vi "0926New Project.vi"() -> ()   [LabVIEW 2011] (continued)
\n7783468750.000000#-39.000000#-4.400000#-18.000000#-10.000000#-3.000000#-30.000000#-30.000000\r\n7789712500.000000#-39.000000#-4.400000#-18.000000#-10.000000#-3.000000#-30.000000#-30.000000\r\n7795956250.000000#-39.000000#-4.400000#-18.000000#-10.000000#-3.000000#-30.000000#-30.000000\r\n7802200000.000000#-39.000000#-4.400000#-18.000000#-10.000000#-3.000000#-30.000000#-30.000000\r\n7808443750.000000#-39.000000#-4.400000#-18.000000#-10.000000#-3.000000#-30.000000#-30.000000\r\n7814687500.000000#-39.000000#-4.400000#-18.000000#-10.000000#-3.000000#-30.000000#-30.000000\r\n7820931250.000000#-39.000000#-4.400000#-18.000000#-10.000000#-3.000000#-30.000000#-30.000000\r\n7827175000.000000#-39.000000#-4.400000#-18.000000#-10.000000#-3.000000#-30.000000#-30.000000\r\n7833418750.000000#-39.000000#-4.400000#-18.000000#-10.000000#-3.000000#-30.000000#-30.000000\r\n7839662500.000000#-39.000000#-4.400000#-18.000000#-10.000000#-3.000000#-30.000000#-30.000000\r\n7845906250.000000#-39.000000#-4.400000#-18.000000#-10.000000#-3.000000#-30.000000#-30.000000\r\n7852150000.000000#-39.000000#-4.400000#-18.000000#-10.000000#-3.000000#-30.000000#-30.000000\r\n7858393750.000000#-39.000000#-4.400000#-18.000000#-10.000000#-3.000000#-30.000000#-30.000000\r\n7864637500.000000#-39.000000#-4.400000#-18.000000#-10.000000#-3.000000#-30.000000#-30.000000\r\n7870881250.000000#-39.000000#-4.400000#-18.000000#-10.000000#-3.000000#-30.000000#-30.000000\r\n7877125000.000000#-39.000000#-4.400000#-18.000000#-10.000000#-3.000000#-30.000000#-30.000000\r\n7883368750.000000#-39.000000#-4.400000#-18.000000#-10.000000#-3.000000#-30.000000#-30.000000\r\n7889612500.000000#-39.000000#-4.400000#-18.000000#-10.000000#-3.000000#-30.000000#-30.000000\r\n7895856250.000000#-39.000000#-4.400000#-18.000000#-10.000000#-3.000000#-30.000000#-30.000000\r\n7902100000.000000#-39.000000#-4.400000#-18.000000#-10.000000#-3.000000#-30.000000#-30.000000\r\n7908343750.000000#-39.000000#-4.400000#-18.000000#-10.000000#-3.000000#-30.000000#-30.000000\r\n7914587500.000000#-39.000000#-4.400000#-18.000000#-10.000000#-3.000000#-30.000000#-30.000000\r\n7920831250.000000#-39.000000#-4.400000#-18.000000#-10.000000#-3.000000#-30.000000#-30.000000\r\n7927075000.000000#-39.000000#-4.400000#-18.000000#-10.000000#-3.000000#-30.000000#-30.000000\r\n7933318750.000000#-39.000000#-4.400000#-18.000000#-10.000000#-3.000000#-30.000000#-30.000000\r\n7939562500.000000#-39.000000#-4.400000#-18.000000#-10.000000#-3.000000#-30.000000#-30.000000\r\n7945806250.000000#-39.000000#-4.400000#-18.000000#-10.000000#-3.000000#-30.000000#-30.000000\r\n7952050000.000000#-39.000000#-4.400000#-18.000000#-10.000000#-3.000000#-30.000000#-30.000000\r\n7958293750.000000#-39.000000#-4.400000#-18.000000#-10.000000#-3.000000#-30.000000#-30.000000\r\n7964537500.000000#-39.000000#-4.400000#-18.000000#-10.000000#-3.000000#-30.000000#-30.000000\r\n7970781250.000000#-39.000000#-4.400000#-18.000000#-10.000000#-3.000000#-30.000000#-30.000000\r\n7977025000.000000#-39.000000#-4.400000#-18.000000#-10.000000#-3.000000#-30.000000#-30.000000\r\n7983268750.000000#-39.000000#-4.400000#-18.000000#-10.000000#-3.000000#-30.000000#-30.000000\r\n7989512500.000000#-39.000000#-4.400000#-18.000000#-10.000000#-3.000000#-30.000000#-30.000000\r\n7995756250.000000#-39.000000#-4.400000#-18.000000#-10.000000#-3.000000#-30.000000#-30.000000\r\n8002000000.000000#-39.000000#-4.400000#-18.000000#-10.000000#-3.000000#-30.000000#-30.000000\r\n8008243750.000000#-39.000000#-4.400000#-18.000000#-10.000000#-3.000000#-30.000000#-30.000000\r\n8014487500.000000#-39.000000#-4.400000#-18.000000#-10.000000#-3.000000#-30.000000#-30.000000\r\n8020731250.000000#-39.000000#-4.400000#-18.000000#-10.000000#-3.000000#-30.000000#-30.000000\r\n8026975000.000000#-39.000000#-4.400000#-18.000000#-10.000000#-3.000000#-30.000000#-30.000000\r\n8033218750.000000#-39.000000#-4.400000#-18.000000#-10.000000#-3.000000#-30.000000#-30.000000\r\n8039462500.000000#-39.000000#-4.400000#-18.000000#-10.000000#-3.000000#-30.000000#-30.000000\r\n8045706250.000000#-39.000000#-4.400000#-18.000000#-10.000000#-3.000000#-30.000000#-30.000000\r\n8051950000.000000#-39.000000#-4.400000#-18.000000#-10.000000#-3.000000#-30.000000#-30.000000\r\n8058193750.000000#-39.000000#-4.400000#-18.000000#-10.000000#-3.000000#-30.000000#-30.000000\r\n8064437500.000000#-39.000000#-4.400000#-18.000000#-10.000000#-3.000000#-30.000000#-30.000000\r\n8070681250.000000#-39.000000#-4.400000#-18.000000#-10.000000#-3.000000#-30.000000#-30.000000\r\n8076925000.000000#-39.000000#-4.400000#-18.000000#-10.000000#-3.000000#-30.000000#-30.000000\r\n8083168750.000000#-39.000000#-4.400000#-18.000000#-10.000000#-3.000000#-30.000000#-30.000000\r\n8089412500.000000#-39.000000#-4.400000#-18.000000#-10.000000#-3.000000#-30.000000#-30.000000\r\n8095656250.000000#-39.000000#-4.400000#-18.000000#-10.000000#-3.000000#-30.000000#-30.000000\r\n8101900000.000000#-39.000000#-4.400000#-18.000000#-10.000000#-3.000000#-30.000000#-30.000000\r\n8108143750.000000#-39.000000#-4.400000#-18.000000#-10.000000#-3.000000#-30.000000#-30.000000\r\n8114387500.000000#-39.000000#-4.400000#-18.000000#-10.000000#-3.000000#-30.000000#-30.000000\r\n8120631250.000000#-39.000000#-4.400000#-18.000000#-10.000000#-3.000000#-30.000000#-30.000000\r\n8126875000.000000#-39.000000#-4.400000#-18.000000#-10.000000#-3.000000#-30.000000#-30.000000\r\n8133118750.000000#-39.000000#-4.400000#-18.000000#-10.000000#-3.000000#-30.000000#-30.000000\r\n8139362500.000000#-39.000000#-4.400000#-18.000000#-10.000000#-3.000000#-30.000000#-30.000000\r\n8145606250.000000#-39.000000#-4.400000#-18.000000#-10.000000#-3.000000#-30.000000#-30.000000\r\n8151850000.000000#-39.000000#-4.400000#-18.000000#-10.000000#-3.000000#-30.000000#-30.000000\r\n8158093750.000000#-39.000000#-4.400000#-18.000000#-10.000000#-3.000000#-30.000000#-30.000000\r\n8164337500.000000#-39.000000#-4.400000#-18.000000#-10.000000#-3.000000#-30.000000#-30.000000\r\n8170581250.000000#-39.000000#-4.400000#-18.000000#-10.000000#-3.000000#-30.000000#-30.000000\r\n8176825000.000000#-39.000000#-4.400000#-18.000000#-10.000000#-3.000000#-30.000000#-30.000000\r\n8183068750.000000#-39.000000#-4.400000#-18.000000#-10.000000#-3.000000#-30.000000#-30.000000\r\n8189312500.000000#-39.000000#-4.400000#-18.000000#-10.000000#-3.000000#-30.000000#-30.000000\r\n8195556250.000000#-39.000000#-4.400000#-18.000000#-10.000000#-3.000000#-30.000000#-30.000000\r\n8201800000.000000#-39.000000#-4.400000#-18.000000#-10.000000#-3.000000#-30.000000#-30.000000\r\n8208043750.000000#-39.000000#-4.400000#-18.000000#-10.000000#-3.000000#-30.000000#-30.000000\r\n8214287500.000000#-39.000000#-4.400000#-18.000000#-10.000000#-3.000000#-30.000000#-30.000000\r\n8220531250.000000#-39.000000#-4.400000#-18.000000#-10.000000#-3.000000#-30.000000#-30.000000\r\n8226775000.000000#-39.000000#-4.400000#-18.000000#-10.000000#-3.000000#-30.000000#-30.000000\r\n8233018750.000000#-39.000000#-4.400000#-18.000000#-10.000000#-3.000000#-30.000000#-30.000000\r\n8239262500.000000#-39.000000#-4.400000#-18.000000#-10.000000#-3.000000#-30.000000#-30.000000\r\n8245506250.000000#-39.000000#-4.400000#-18.000000#-10.000000#-3.000000#-30.000000#-30.000000\r\n8251750000.000000#-39.000000#-4.400000#-18.000000#-10.000000#-3.000000#-30.000000#-30.000000\r\n8257993750.000000#-39.000000#-4.400000#-18.000000#-10.000000#-3.000000#-30.000000#-30.000000\r\n8264237500.000000#-39.000000#-4.400000#-18.000000#-10.000000#-3.000000#-30.000000#-30.000000\r\n8270481250.000000#-39.000000#-4.400000#-18.000000#-10.000000#-3.000000#-30.000000#-30.000000\r\n8276725000.000000#-39.000000#-4.400000#-18.000000#-10.000000#-3.000000#-30.000000#-30.000000\r\n8282968750.000000#-39.000000#-4.400000#-18.000000#-10.000000#-3.000000#-30.000000#-30.000000\r\n8289212500.000000#-39.000000#-4.400000#-18.000000#-10.000000#-3.000000#-30.000000#-30.000000\r\n8295456250.000000#-39.000000#-4.400000#-18.000000#-10.000000#-3.000000#-30.000000#-30.000000\r\n8301700000.000000#-39.000000#-4.400000#-18.000000#-10.000000#-3.000000#-30.000000#-30.000000\r\n8307943750.000000#-39.000000#-4.400000#-18.000000#-10.000000#-3.000000#-30.000000#-30.000000\r\n8314187500.000000#-39.000000#-4.400000#-18.000000#-10.000000#-3.000000#-30.000000#-30.000000\r\n8320431250.000000#-39.000000#-4.400000#-18.000000#-10.000000#-3.000000#-30.000000#-30.000000\r\n8326675000.000000#-39.000000#-4.400000#-18.000000#-10.000000#-3.000000#-30.000000#-30.000000\r\n8332918750.000000#-39.000000#-4.400000#-18.000000#-10.000000#-3.000000#-30.000000#-30.000000\r\n8339162500.000000#-39.000000#-4.400000#-18.000000#-10.000000#-3.000000#-30.000000#-30.000000\r\n8345406250.000000#-39.000000#-4.400000#-18.000000#-10.000000#-3.000000#-30.000000#-30.000000\r\n8351650000.000000#-39.000000#-4.400000#-18.000000#-10.000000#-3.000000#-30.000000#-30.000000\r\n8357893750.000000#-39.000000#-4.400000#-18.000000#-10.000000#-3.000000#-30.000000#-30.000000\r\n8364137500.000000#-39.000000#-4.400000#-18.000000#-10.000000#-3.000000#-30.000000#-30.000000\r\n8370381250.000000#-39.000000#-4.400000#-18.000000#-10.000000#-3.000000#-30.000000#-30.000000\r\n8376625000.000000#-39.000000#-4.400000#-18.000000#-10.000000#-3.000000#-30.000000#-30.000000\r\n8382868750.000000#-39.000000#-4.400000#-18.000000#-10.000000#-3.000000#-30.000000#-30.000000\r\n8389112500.000000#-39.000000#-4.400000#-18.000000#-10.000000#-3.000000#-30.000000#-30.000000\r\n8395356250.000000#-39.000000#-4.400000#-18.000000#-10.000000#-3.000000#-30.000000#-30.000000\r\n8401600000.000000#-39.000000#-4.400000#-18.000000#-10.000000#-3.000000#-30.000000#-30.000000\r\n8407843750.000000#-39.000000#-4.400000#-18.000000#-10.000000#-3.000000#-30.000000#-30.000000\r\n8414087500.000000#-39.000000#-4.400000#-18.000000#-10.000000#-3.000000#-30.000000#-30.000000\r\n8420331250.000000#-39.000000#-4.400000#-18.000000#-10.000000#-3.000000#-30.000000#-30.000000\r\n8426575000.000000#-39.000000#-4.400000#-18.000000#-10.000000#-3.000000#-30.000000#-30.000000\r\n8432818750.000000#-39.000000#-4.400000#-18.000000#-10.000000#-3.000000#-30.000000#-30.000000\r\n8439062500.000000#-39.000000#-4.400000#-18.000000#-10.000000#-3.000000#-30.000000#-30.000000\r\n8445306250.000000#-39.000000#-4.400000#-18.000000#-10.000000#-3.000000#-30.000000#-30.000000\r\n8451550000.000000#-39.000000#-4.400000#-18.000000#-10.000000#-3.000000#-30.000000#-30.000000\r\n8457793750.000000#-39.000000#-4.400000#-18.000000#-10.000000#-3.000000#-30.000000#-30.000000\r\n8464037500.000000#-39.000000#-4.400000#-18.000000#-10.000000#-3.000000#-30.000000#-30.000000\r\n8470281250.000000#-39.000000#-4.400000#-18.000000#-10.000000#-3.000000#-30.000000#-30.000000\r\n8476525000.000000#-39.000000#-4.400000#-18.000000#-10.000000#-3.000000#-30.000000#-30.000000\r\n8482768750.000000#-39.000000#-4.400000#-18.000000#-10.000000#-3.000000#-30.000000#-30.000000\r\n8489012500.000000#-39.000000#-4.400000#-18.000000#-10.000000#-3.000000#-30.000000#-30.000000\r\n8495256250.000000#-39.000000#-4.400000#-18.000000#-10.000000#-3.000000#-30.000000#-30.000000\r\n8501500000.000000#-39.000000#-4.400000#-18.000000#-10.000000#-3.000000#-30.000000#-30.000000\r\n8507743750.000000#-39.000000#-4.400000#-18.000000#-10.000000#-3.000000#-30.000000#-30.000000\r\n8513987500.000000#-39.000000#-4.400000#-18.000000#-10.000000#-3.000000#-30.000000#-30.000000\r\n8520231250.000000#-39.000000#-4.400000#-18.000000#-10.000000#-3.000000#-30.000000#-30.000000\r\n8526475000.000000#-39.000000#-4.400000#-18.000000#-10.000000#-3.000000#-30.000000#-30.000000\r\n8532718750.000000#-39.000000#-4.400000#-18.000000#-10.000000#-3.000000#-30.000000#-30.000000\r\n8538962500.000000#-39.000000#-4.400000#-18.000000#-10.000000#-3.000000#-30.000000#-30.000000\r\n8545206250.000000#-39.000000#-4.400000#-18.000000#-10.000000#-3.000000#-30.000000#-30.000000\r\n8551450000.000000#-39.000000#-4.400000#-18.000000#-10.000000#-3.000000#-30.000000#-30.000000\r\n8557693750.000000#-39.000000#-4.400000#-18.000000#-10.000000#-3.000000#-30.000000#-30.000000\r\n8563937500.000000#-39.000000#-4.400000#-18.000000#-10.000000#-3.000000#-30.000000#-30.000000\r\n8570181250.000000#-39.000000#-4.400000#-18.000000#-10.000000#-3.000000#-30.000000#-30.000000\r\n8576425000.000000#-39.000000#-4.400000#-18.000000#-10.000000#-3.000000#-30.000000#-30.000000\r\n8582668750.000000#-39.000000#-4.400000#-18.000000#-10.000000#-3.000000#-30.000000#-30.000000\r\n8588912500.000000#-39.000000#-4.400000#-18.000000#-10.000000#-3.000000#-30.000000#-30.000000\r\n8595156250.000000#-39.000000#-4.400000#-18.000000#-10.000000#-3.000000#-30.000000#-30.000000\r\n8601400000.000000#-39.000000#-4.400000#-18.000000#-10.000000#-3.000000#-30.000000#-30.000000\r\n8607643750.000000#-39.000000#-4.400000#-18.000000#-10.000000#-3.000000#-30.000000#-30.000000\r\n8613887500.000000#-39.000000#-4.400000#-18.000000#-10.000000#-3.000000#-30.000000#-30.000000\r\n8620131250.000000#-39.000000#-4.400000#-18.000000#-10.000000#-3.000000#-30.000000#-30.000000\r\n8626375000.000000#-39.000000#-4.400000#-18.000000#-10.000000#-3.000000#-30.000000#-30.000000\r\n8632618750.000000#-39.000000#-4.400000#-18.000000#-10.000000#-3.000000#-30.000000#-30.000000\r\n8638862500.000000#-39.000000#-4.400000#-18.000000#-10.000000#-3.000000#-30.000000#-30.000000\r\n8645106250.000000#-39.000000#-4.400000#-18.000000#-10.000000#-3.000000#-30.000000#-30.000000\r\n8651350000.000000#-39.000000#-4.400000#-18.000000#-10.000000#-3.000000#-30.000000#-30.000000\r\n8657593750.000000#-39.000000#-4.400000#-18.000000#-10.000000#-3.000000#-30.000000#-30.000000\r\n8663837500.000000#-39.000000#-4.400000#-18.000000#-10.000000#-3.000000#-30.000000#-30.000000\r\n8670081250.000000#-39.000000#-4.400000#-18.000000#-10.000000#-3.000000#-30.000000#-30.000000\r\n8676325000.000000#-39.000000#-4.400000#-18.000000#-10.000000#-3.000000#-30.000000#-30.000000\r\n8682568750.000000#-39.000000#-4.400000#-18.000000#-10.000000#-3.000000#-30.000000#-30.000000\r\n8688812500.000000#-39.000000#-4.400000#-18.000000#-10.000000#-3.000000#-30.000000#-30.000000\r\n8695056250.000000#-39.000000#-4.400000#-18.000000#-10.000000#-3.000000#-30.000000#-30.000000\r\n8701300000.000000#-39.000000#-4.400000#-18.000000#-10.000000#-3.000000#-30.000000#-30.000000\r\n8707543750.000000#-39.000000#-4.400000#-18.000000#-10.000000#-3.000000#-30.000000#-30.000000\r\n8713787500.000000#-39.000000#-4.400000#-18.000000#-10.000000#-3.000000#-30.000000#-30.000000\r\n8720031250.000000#-39.000000#-4.400000#-18.000000#-10.000000#-3.000000#-30.000000#-30.000000\r\n8726275000.000000#-39.000000#-4.400000#-18.000000#-10.000000#-3.000000#-30.000000#-30.000000\r\n8732518750.000000#-39.000000#-4.400000#-18.000000#-10.000000#-3.000000#-30.000000#-30.000000\r\n8738762500.000000#-39.000000#-4.400000#-18.000000#-10.000000#-3.000000#-30.000000#-30.000000\r\n8745006250.000000#-39.000000#-4.400000#-18.000000#-10.000000#-3.000000#-30.000000#-30.000000\r\n8751250000.000000#-39.000000#-4.400000#-18.000000#-10.000000#-3.000000#-30.000000#-30.000000\r\n8757493750.000000#-39.000000#-4.400000#-18.000000#-10.000000#-3.000000#-30.000000#-30.000000\r\n8763737500.000000#-39.000000#-4.400000#-18.000000#-10.000000#-3.000000#-30.000000#-30.000000\r\n8769981250.000000#-39.000000#-4.400000#-18.000000#-10.000000#-3.000000#-30.000000#-30.000000\r\n8776225000.000000#-39.000000#-4.400000#-18.000000#-10.000000#-3.000000#-30.000000#-30.000000\r\n8782468750.000000#-39.000000#-4.400000#-18.000000#-10.000000#-3.000000#-30.000000#-30.000000\r\n8788712500.000000#-39.000000#-4.400000#-18.000000#-10.000000#-3.000000#-30.000000#-30.000000\r\n8794956250.000000#-39.000000#-4.400000#-18.000000#-10.000000#-3.000000#-30.000000#-30.000000\r\n8801200000.000000#-39.000000#-4.400000#-18.000000#-10.000000#-3.000000#-30.000000#-30.000000\r\n8807443750.000000#-39.000000#-4.400000#-18.000000#-10.000000#-3.000000#-30.000000#-30.000000\r\n8813687500.000000#-39.000000#-4.400000#-18.000000#-10.000000#-3.000000#-30.000000#-30.000000\r\n8819931250.000000#-39.000000#-4.400000#-18.000000#-10.000000#-3.000000#-30.000000#-30.000000\r\n8826175000.000000#-39.000000#-4.400000#-18.000000#-10.000000#-3.000000#-30.000000#-30.000000\r\n8832418750.000000#-39.000000#-4.400000#-18.000000#-10.000000#-3.000000#-30.000000#-30.000000\r\n8838662500.000000#-39.000000#-4.400000#-18.000000#-10.000000#-3.000000#-30.000000#-30.000000\r\n8844906250.000000#-39.000000#-4.400000#-18.000000#-10.000000#-3.000000#-30.000000#-30.000000\r\n8851150000.000000#-39.000000#-4.400000#-18.000000#-10.000000#-3.000000#-30.000000#-30.000000\r\n8857393750.000000#-39.000000#-4.400000#-18.000000#-10.000000#-3.000000#-30.000000#-30.000000\r\n8863637500.000000#-39.000000#-4.400000#-18.000000#-10.000000#-3.000000#-30.000000#-30.000000\r\n8869881250.000000#-39.000000#-4.400000#-18.000000#-10.000000#-3.000000#-30.000000#-30.000000\r\n8876125000.000000#-39.000000#-4.400000#-18.000000#-10.000000#-3.000000#-30.000000#-30.000000\r\n8882368750.000000#-39.000000#-4.400000#-18.000000#-10.000000#-3.000000#-30.000000#-30.000000\r\n8888612500.000000#-39.000000#-4.400000#-18.000000#-10.000000#-3.000000#-30.000000#-30.000000\r\n8894856250.000000#-39.000000#-4.400000#-18.000000#-10.000000#-3.000000#-30.000000#-30.000000\r\n8901100000.000000#-39.000000#-4.400000#-18.000000#-10.000000#-3.000000#-30.000000#-30.000000\r\n8907343750.000000#-39.000000#-4.400000#-18.000000#-10.000000#-3.000000#-30.000000#-30.000000\r\n8913587500.000000#-39.000000#-4.400000#-18.000000#-10.000000#-3.000000#-30.000000#-30.000000\r\n8919831250.000000#-39.000000#-4.400000#-18.000000#-10.000000#-3.000000#-30.000000#-30.000000\r\n8926075000.000000#-39.000000#-4.400000#-18.000000#-10.000000#-3.000000#-30.000000#-30.000000\r\n8932318750.000000#-39.000000#-4.400000#-18.000000#-10.000000#-3.000000#-30.000000#-30.000000\r\n8938562500.000000#-39.000000#-4.400000#-18.000000#-10.000000#-3.000000#-30.000000#-30.000000\r\n8944806250.000000#-39.000000#-4.400000#-18.000000#-10.000000#-3.000000#-30.000000#-30.000000\r\n8951050000.000000#-39.000000#-4.400000#-18.000000#-10.000000#-3.000000#-30.000000#-30.000000\r\n8957293750.000000#-39.000000#-4.400000#-18.000000#-10.000000#-3.000000#-30.000000#-30.000000\r\n8963537500.000000#-39.000000#-4.400000#-18.000000#-10.000000#-3.000000#-30.000000#-30.000000\r\n8969781250.000000#-39.000000#-4.400000#-18.000000#-10.000000#-3.000000#-30.000000#-30.000000\r\n8976025000.000000#-39.000000#-4.400000#-18.000000#-10.000000#-3.000000#-30.000000#-30.000000\r\n8982268750.000000#-39.000000#-4.400000#-18.000000#-10.000000#-3.000000#-30.000000#-30.000000\r\n8988512500.000000#-39.000000#-4.400000#-18.000000#-10.000000#-3.000000#-30.000000#-30.000000\r\n8994756250.000000#-39.000000#-4.400000#-18.000000#-10.000000#-3.000000#-30.000000#-30.000000\r\n9001000000.000000#-39.000000#-4.400000#-18.000000#-10.000000#-3.000000#-30.000000#-30.000000\r\n9007243750.000000#-39.000000#-3.500000#-18.000000#-10.000000#-3.000000#-30.000000#-30.000000\r\n9013487500.000000#-39.000000#-3.500000#-18.000000#-10.000000#-3.000000#-30.000000#-30.000000\r\n9019731250.000000#-39.000000#-3.500000#-18.000000#-10.000000#-3.000000#-30.000000#-30.000000\r\n9025975000.000000#-39.000000#-3.500000#-18.000000#-10.000000#-3.000000#-30.000000#-30.000000\r\n9032218750.000000#-39.000000#-3.500000#-18.000000#-10.000000#-3.000000#-30.000000#-30.000000\r\n9038462500.000000#-39.000000#-3.500000#-18.000000#-10.000000#-3.000000#-30.000000#-30.000000\r\n9044706250.000000#-39.000000#-3.500000#-18.000000#-10.000000#-3.000000#-30.000000#-30.000000\r\n9050950000.000000#-39.000000#-3.500000#-18.000000#-10.000000#-3.000000#-30.000000#-30.000000\r\n9057193750.000000#-39.000000#-3.500000#-18.000000#-10.000000#-3.000000#-30.000000#-30.000000\r\n9063437500.000000#-39.000000#-3.500000#-18.000000#-10.000000#-3.000000#-30.000000#-30.000000\r\n9069681250.000000#-39.000000#-3.500000#-18.000000#-10.000000#-3.000000#-30.000000#-30.000000\r\n9075925000.000000#-39.000000#-3.500000#-18.000000#-10.000000#-3.000000#-30.000000#-30.000000\r\n9082168750.000000#-39.000000#-3.500000#-18.000000#-10.000000#-3.000000#-30.000000#-30.000000\r\n9088412500.000000#-39.000000#-3.500000#-18.000000#-10.000000#-3.000000#-30.000000#-30.000000\r\n9094656250.000000#-39.000000#-3.500000#-18.000000#-10.000000#-3.000000#-30.000000#-30.000000\r\n9100900000.000000#-39.000000#-3.500000#-18.000000#-10.000000#-3.000000#-30.000000#-30.000000\r\n9107143750.000000#-39.000000#-3.500000#-18.000000#-10.000000#-3.000000#-30.000000#-30.000000\r\n9113387500.000000#-39.000000#-3.500000#-18.000000#-10.000000#-3.000000#-30.000000#-30.000000\r\n9119631250.000000#-39.000000#-3.500000#-18.000000#-10.000000#-3.000000#-30.000000#-30.000000\r\n9125875000.000000#-39.000000#-3.500000#-18.000000#-10.000000#-3.000000#-30.000000#-30.000000\r\n9132118750.000000#-39.000000#-3.500000#-18.000000#-10.000000#-3.000000#-30.000000#-30.000000\r\n9138362500.000000#-39.000000#-3.500000#-18.000000#-10.000000#-3.000000#-30.000000#-30.000000\r\n9144606250.000000#-39.000000#-3.500000#-18.000000#-10.000000#-3.000000#-30.000000#-30.000000\r\n9150850000.000000#-39.000000#-3.500000#-18.000000#-10.000000#-3.000000#-30.000000#-30.000000\r\n9157093750.000000#-39.000000#-3.500000#-18.000000#-10.000000#-3.000000#-30.000000#-30.000000\r\n9163337500.000000#-39.000000#-3.500000#-18.000000#-10.000000#-3.000000#-30.000000#-30.000000\r\n9169581250.000000#-39.000000#-3.500000#-18.000000#-10.000000#-3.000000#-30.000000#-30.000000\r\n9175825000.000000#-39.000000#-3.500000#-18.000000#-10.000000#-3.000000#-30.000000#-30.000000\r\n9182068750.000000#-39.000000#-3.500000#-18.000000#-10.000000#-3.000000#-30.000000#-30.000000\r\n9188312500.000000#-39.000000#-3.500000#-18.000000#-10.000000#-3.000000#-30.000000#-30.000000\r\n9194556250.000000#-39.000000#-3.500000#-18.000000#-10.000000#-3.000000#-30.000000#-30.000000\r\n9200800000.000000#-39.000000#-3.500000#-18.000000#-10.000000#-3.000000#-30.000000#-30.000000\r\n9207043750.000000#-39.000000#-3.500000#-18.000000#-10.000000#-3.000000#-30.000000#-30.000000\r\n9213287500.000000#-39.000000#-3.500000#-18.000000#-10.000000#-3.000000#-30.000000#-30.000000\r\n9219531250.000000#-39.000000#-3.500000#-18.000000#-10.000000#-3.000000#-30.000000#-30.000000\r\n9225775000.000000#-39.000000#-3.500000#-18.000000#-10.000000#-3.000000#-30.000000#-30.000000\r\n9232018750.000000#-39.000000#-3.500000#-18.000000#-10.000000#-3.000000#-30.000000#-30.000000\r\n9238262500.000000#-39.000000#-3.500000#-18.000000#-10.000000#-3.000000#-30.000000#-30.000000\r\n9244506250.000000#-39.000000#-3.500000#-18.000000#-10.000000#-3.000000#-30.000000#-30.000000\r\n9250750000.000000#-39.000000#-3.500000#-18.000000#-10.000000#-3.000000#-30.000000#-30.000000\r\n9256993750.000000#-39.000000#-3.500000#-18.000000#-10.000000#-3.000000#-30.000000#-30.000000\r\n9263237500.000000#-39.000000#-3.500000#-18.000000#-10.000000#-3.000000#-30.000000#-30.000000\r\n9269481250.000000#-39.000000#-3.500000#-18.000000#-10.000000#-3.000000#-30.000000#-30.000000\r\n9275725000.000000#-39.000000#-3.500000#-18.000000#-10.000000#-3.000000#-30.000000#-30.000000\r\n9281968750.000000#-39.000000#-3.500000#-18.000000#-10.000000#-3.000000#-30.000000#-30.000000\r\n9288212500.000000#-39.000000#-3.500000#-18.000000#-10.000000#-3.000000#-30.000000#-30.000000\r\n9294456250.000000#-39.000000#-3.500000#-18.000000#-10.000000#-3.000000#-30.000000#-30.000000\r\n9300700000.000000#-39.000000#-3.500000#-18.000000#-10.000000#-3.000000#-30.000000#-30.000000\r\n9306943750.000000#-39.000000#-3.500000#-18.000000#-10.000000#-3.000000#-30.000000#-30.000000\r\n9313187500.000000#-39.000000#-3.500000#-18.000000#-10.000000#-3.000000#-30.000000#-30.000000\r\n9319431250.000000#-39.000000#-3.500000#-18.000000#-10.000000#-3.000000#-30.000000#-30.000000\r\n9325675000.000000#-39.000000#-3.500000#-18.000000#-10.000000#-3.000000#-30.000000#-30.000000\r\n9331918750.000000#-39.000000#-3.500000#-18.000000#-10.000000#-3.000000#-30.000000#-30.000000\r\n9338162500.000000#-39.000000#-3.500000#-18.000000#-10.000000#-3.000000#-30.000000#-30.000000\r\n9344406250.000000#-39.000000#-3.500000#-18.000000#-10.000000#-3.000000#-30.000000#-30.000000\r\n9350650000.000000#-39.000000#-3.500000#-18.000000#-10.000000#-3.000000#-30.000000#-30.000000\r\n9356893750.000000#-39.000000#-3.500000#-18.000000#-10.000000#-3.000000#-30.000000#-30.000000\r\n9363137500.000000#-39.000000#-3.500000#-18.000000#-10.000000#-3.000000#-30.000000#-30.000000\r\n9369381250.000000#-39.000000#-3.500000#-18.000000#-10.000000#-3.000000#-30.000000#-30.000000\r\n9375625000.000000#-39.000000#-3.500000#-18.000000#-10.000000#-3.000000#-30.000000#-30.000000\r\n9381868750.000000#-39.000000#-3.500000#-18.000000#-10.000000#-3.000000#-30.000000#-30.000000\r\n9388112500.000000#-39.000000#-3.500000#-18.000000#-10.000000#-3.000000#-30.000000#-30.000000\r\n9394356250.000000#-39.000000#-3.500000#-18.000000#-10.000000#-3.000000#-30.000000#-30.000000\r\n9400600000.000000#-39.000000#-3.500000#-18.000000#-10.000000#-3.000000#-30.000000#-30.000000\r\n9406843750.000000#-39.000000#-3.500000#-18.000000#-10.000000#-3.000000#-30.000000#-30.000000\r\n9413087500.000000#-39.000000#-3.500000#-18.000000#-10.000000#-3.000000#-30.000000#-30.000000\r\n9419331250.000000#-39.000000#-3.500000#-18.000000#-10.000000#-3.000000#-30.000000#-30.000000\r\n9425575000.000000#-39.000000#-3.500000#-18.000000#-10.000000#-3.000000#-30.000000#-30.000000\r\n9431818750.000000#-39.000000#-3.500000#-18.000000#-10.000000#-3.000000#-30.000000#-30.000000\r\n9438062500.000000#-39.000000#-3.500000#-18.000000#-10.000000#-3.000000#-30.000000#-30.000000\r\n9444306250.000000#-39.000000#-3.500000#-18.000000#-10.000000#-3.000000#-30.000000#-30.000000\r\n9450550000.000000#-39.000000#-3.500000#-18.000000#-10.000000#-3.000000#-30.000000#-30.000000\r\n9456793750.000000#-39.000000#-3.500000#-18.000000#-10.000000#-3.000000#-30.000000#-30.000000\r\n9463037500.000000#-39.000000#-3.500000#-18.000000#-10.000000#-3.000000#-30.000000#-30.000000\r\n9469281250.000000#-39.000000#-3.500000#-18.000000#-10.000000#-3.000000#-30.000000#-30.000000\r\n9475525000.000000#-39.000000#-3.500000#-18.000000#-10.000000#-3.000000#-30.000000#-30.000000\r\n9481768750.000000#-39.000000#-3.500000#-18.000000#-10.000000#-3.000000#-30.000000#-30.000000\r\n9488012500.000000#-39.000000#-3.500000#-18.000000#-10.000000#-3.000000#-30.000000#-30.000000\r\n9494256250.000000#-39.000000#-3.500000#-18.000000#-10.000000#-3.000000#-30.000000#-30.000000\r\n9500500000.000000#-39.000000#-3.500000#-18.000000#-10.000000#-3.000000#-30.000000#-30.000000\r\n9506743750.000000#-39.000000#-3.500000#-18.000000#-10.000000#-3.000000#-30.000000#-30.000000\r\n9512987500.000000#-39.000000#-3.500000#-18.000000#-10.000000#-3.000000#-30.000000#-30.000000\r\n9519231250.000000#-39.000000#-3.500000#-18.000000#-10.000000#-3.000000#-30.000000#-30.000000\r\n9525475000.000000#-39.000000#-3.500000#-18.000000#-10.000000#-3.000000#-30.000000#-30.000000\r\n9531718750.000000#-39.000000#-3.500000#-18.000000#-10.000000#-3.000000#-30.000000#-30.000000\r\n9537962500.000000#-39.000000#-3.500000#-18.000000#-10.000000#-3.000000#-30.000000#-30.000000\r\n9544206250.000000#-39.000000#-3.500000#-18.000000#-10.000000#-3.000000#-30.000000#-30.000000\r\n9550450000.000000#-39.000000#-3.500000#-18.000000#-10.000000#-3.000000#-30.000000#-30.000000\r\n9556693750.000000#-39.000000#-3.500000#-18.000000#-10.000000#-3.000000#-30.000000#-30.000000\r\n9562937500.000000#-39.000000#-3.500000#-18.000000#-10.000000#-3.000000#-30.000000#-30.000000\r\n9569181250.000000#-39.000000#-3.500000#-18.000000#-10.000000#-3.000000#-30.000000#-30.000000\r\n9575425000.000000#-39.000000#-3.500000#-18.000000#-10.000000#-3.000000#-30.000000#-30.000000\r\n9581668750.000000#-39.000000#-3.500000#-18.000000#-10.000000#-3.000000#-30.000000#-30.000000\r\n9587912500.000000#-39.000000#-3.500000#-18.000000#-10.000000#-3.000000#-30.000000#-30.000000\r\n9594156250.000000#-39.000000#-3.500000#-18.000000#-10.000000#-3.000000#-30.000000#-30.000000\r\n9600400000.000000#-39.000000#-3.500000#-18.000000#-10.000000#-3.000000#-30.000000#-30.000000\r\n9606643750.000000#-39.000000#-3.500000#-18.000000#-10.000000#-3.000000#-30.000000#-30.000000\r\n9612887500.000000#-39.000000#-3.500000#-18.000000#-10.000000#-3.000000#-30.000000#-30.000000\r\n9619131250.000000#-39.000000#-3.500000#-18.000000#-10.000000#-3.000000#-30.000000#-30.000000\r\n9625375000.000000#-39.000000#-3.500000#-18.000000#-10.000000#-3.000000#-30.000000#-30.000000\r\n9631618750.000000#-39.000000#-3.500000#-18.000000#-10.000000#-3.000000#-30.000000#-30.000000\r\n9637862500.000000#-39.000000#-3.500000#-18.000000#-10.000000#-3.000000#-30.000000#-30.000000\r\n9644106250.000000#-39.000000#-3.500000#-18.000000#-10.000000#-3.000000#-30.000000#-30.000000\r\n9650350000.000000#-39.000000#-3.500000#-18.000000#-10.000000#-3.000000#-30.000000#-30.000000\r\n9656593750.000000#-39.000000#-3.500000#-18.000000#-10.000000#-3.000000#-30.000000#-30.000000\r\n9662837500.000000#-39.000000#-3.500000#-18.000000#-10.000000#-3.000000#-30.000000#-30.000000\r\n9669081250.000000#-39.000000#-3.500000#-18.000000#-10.000000#-3.000000#-30.000000#-30.000000\r\n9675325000.000000#-39.000000#-3.500000#-18.000000#-10.000000#-3.000000#-30.000000#-30.000000\r\n9681568750.000000#-39.000000#-3.500000#-18.000000#-10.000000#-3.000000#-30.000000#-30.000000\r\n9687812500.000000#-39.000000#-3.500000#-18.000000#-10.000000#-3.000000#-30.000000#-30.000000\r\n9694056250.000000#-39.000000#-3.500000#-18.000000#-10.000000#-3.000000#-30.000000#-30.000000\r\n9700300000.000000#-39.000000#-3.500000#-18.000000#-10.000000#-3.000000#-30.000000#-30.000000\r\n9706543750.000000#-39.000000#-3.500000#-18.000000#-10.000000#-3.000000#-30.000000#-30.000000\r\n9712787500.000000#-39.000000#-3.500000#-18.000000#-10.000000#-3.000000#-30.000000#-30.000000\r\n9719031250.000000#-39.000000#-3.500000#-18.000000#-10.000000#-3.000000#-30.000000#-30.000000\r\n9725275000.000000#-39.000000#-3.500000#-18.000000#-10.000000#-3.000000#-30.000000#-30.000000\r\n9731518750.000000#-39.000000#-3.500000#-18.000000#-10.000000#-3.000000#-30.000000#-30.000000\r\n9737762500.000000#-39.000000#-3.500000#-18.000000#-10.000000#-3.000000#-30.000000#-30.000000\r\n9744006250.000000#-39.000000#-3.500000#-18.000000#-10.000000#-3.000000#-30.000000#-30.000000\r\n9750250000.000000#-39.000000#-3.500000#-18.000000#-10.000000#-3.000000#-30.000000#-30.000000\r\n9756493750.000000#-39.000000#-3.500000#-18.000000#-10.000000#-3.000000#-30.000000#-30.000000\r\n9762737500.000000#-39.000000#-3.500000#-18.000000#-10.000000#-3.000000#-30.000000#-30.000000\r\n9768981250.000000#-39.000000#-3.500000#-18.000000#-10.000000#-3.000000#-30.000000#-30.000000\r\n9775225000.000000#-39.000000#-3.500000#-18.000000#-10.000000#-3.000000#-30.000000#-30.000000\r\n9781468750.000000#-39.000000#-3.500000#-18.000000#-10.000000#-3.000000#-30.000000#-30.000000\r\n9787712500.000000#-39.000000#-3.500000#-18.000000#-10.000000#-3.000000#-30.000000#-30.000000\r\n9793956250.000000#-39.000000#-3.500000#-18.000000#-10.000000#-3.000000#-30.000000#-30.000000\r\n9800200000.000000#-39.000000#-3.500000#-18.000000#-10.000000#-3.000000#-30.000000#-30.000000\r\n9806443750.000000#-39.000000#-3.500000#-18.000000#-10.000000#-3.000000#-30.000000#-30.000000\r\n9812687500.000000#-39.000000#-3.500000#-18.000000#-10.000000#-3.000000#-30.000000#-30.000000\r\n9818931250.000000#-39.000000#-3.500000#-18.000000#-10.000000#-3.000000#-30.000000#-30.000000\r\n9825175000.000000#-39.000000#-3.500000#-18.000000#-10.000000#-3.000000#-30.000000#-30.000000\r\n9831418750.000000#-39.000000#-3.500000#-18.000000#-10.000000#-3.000000#-30.000000#-30.000000\r\n9837662500.000000#-39.000000#-3.500000#-18.000000#-10.000000#-3.000000#-30.000000#-30.000000\r\n9843906250.000000#-39.000000#-3.500000#-18.000000#-10.000000#-3.000000#-30.000000#-30.000000\r\n9850150000.000000#-39.000000#-3.500000#-18.000000#-10.000000#-3.000000#-30.000000#-30.000000\r\n9856393750.000000#-39.000000#-3.500000#-18.000000#-10.000000#-3.000000#-30.000000#-30.000000\r\n9862637500.000000#-39.000000#-3.500000#-18.000000#-10.000000#-3.000000#-30.000000#-30.000000\r\n9868881250.000000#-39.000000#-3.500000#-18.000000#-10.000000#-3.000000#-30.000000#-30.000000\r\n9875125000.000000#-39.000000#-3.500000#-18.000000#-10.000000#-3.000000#-30.000000#-30.000000\r\n9881368750.000000#-39.000000#-3.500000#-18.000000#-10.000000#-3.000000#-30.000000#-30.000000\r\n9887612500.000000#-39.000000#-3.500000#-18.000000#-10.000000#-3.000000#-30.000000#-30.000000\r\n9893856250.000000#-39.000000#-3.500000#-18.000000#-10.000000#-3.000000#-30.000000#-30.000000\r\n9900100000.000000#-39.000000#-3.500000#-18.000000#-10.000000#-3.000000#-30.000000#-30.000000\r\n9906343750.000000#-39.000000#-3.500000#-18.000000#-10.000000#-3.000000#-30.000000#-30.000000\r\n9912587500.000000#-39.000000#-3.500000#-18.000000#-10.000000#-3.000000#-30.000000#-30.000000\r\n9918831250.000000#-39.000000#-3.500000#-18.000000#-10.000000#-3.000000#-30.000000#-30.000000\r\n9925075000.000000#-39.000000#-3.500000#-18.000000#-10.000000#-3.000000#-30.000000#-30.000000\r\n9931318750.000000#-39.000000#-3.500000#-18.000000#-10.000000#-3.000000#-30.000000#-30.000000\r\n9937562500.000000#-39.000000#-3.500000#-18.000000#-10.000000#-3.000000#-30.000000#-30.000000\r\n9943806250.000000#-39.000000#-3.500000#-18.000000#-10.000000#-3.000000#-30.000000#-30.000000\r\n9950050000.000000#-39.000000#-3.500000#-18.000000#-10.000000#-3.000000#-30.000000#-30.000000\r\n9956293750.000000#-39.000000#-3.500000#-18.000000#-10.000000#-3.000000#-30.000000#-30.000000\r\n9962537500.000000#-39.000000#-3.500000#-18.000000#-10.000000#-3.000000#-30.000000#-30.000000\r\n9968781250.000000#-39.000000#-3.500000#-18.000000#-10.000000#-3.000000#-30.000000#-30.000000\r\n9975025000.000000#-39.000000#-3.500000#-18.000000#-10.000000#-3.000000#-30.000000#-30.000000\r\n9981268750.000000#-39.000000#-3.500000#-18.000000#-10.000000#-3.000000#-30.000000#-30.000000\r\n9987512500.000000#-39.000000#-3.500000#-18.000000#-10.000000#-3.000000#-30.000000#-30.000000\r\n9993756250.000000#-39.000000#-3.500000#-18.000000#-10.000000#-3.000000#-30.000000#-30.000000\r\nNaN#NaN#NaN#NaN#NaN#NaN#NaN#NaN\r\n"
  out "Inf":string[][](array[string])=[["SDD21", "S11", "TDD11", "TX1", "TX1-RX1", "TX2-RX1", "Wave Zhang", "Chenhui Zeng"], ["SDD12", "S12", "TDD22", "RX1", "TX2-RX1", "TX3-RX1", "Longjun Zhou", "Jet Shen"], ["SDD11", "S13", "TDD12", "TX2", "TX3-RX1", "TX4-RX1", "Hui Pan", ""], ["SDD22", "S14", "TDD21", "RX2", "TX4-RX1", "TX1-RX2", "Lindsay Gu", ""], ["SCD21", "S21", "TCC11", "TX3", "TX1-RX2", "TX3-RX2", "Xiaoyue Xiang", ""], ["SCD12", "S22", "TCC22", "RX3", "TX2-RX2", "TX4-RX2", "Fenglian Shi", ""], ["SCD22", "S23", "T11", "TX4", "TX3-RX2", "TX1-RX3", "", ""], ["SCD11", "S24", "T22", "RX4", "TX4-RX2", "TX2-RX3", "", ""], ["SDC11", "S31", "T33", "TX5", "TX1-RX3", "TX4-RX3", "", ""], ["SDC22", "S32", "T44", "RX5", "TX2-RX3", "TX1-RX4", "", ""], ["SDC12", "S33", "T12", "TX6", "TX3-RX3", "TX2-RX4", "", ""], ["SDC21", "S34", "T34", "RX6", "TX4-RX3", "TX3-RX4", "", ""], ["SCC11", "S41", "T13", "TX7", "TX1-RX4", "", "", ""], ["SCC22", "S42", "T24", "RX7", "TX2-RX4", "", "", ""], ["SCC12", "S43", "Pskew", "TX8", "TX3-RX4", "", "", ""], ["SCC21", "S44", "", "RX8", "TX4-RX4", "", "", ""], ["SCD21-SDD21", "", "", "", "", "", "", ""], ["ILD", "", "", "", "", "", "", ""], ["NEXT", "", "", "", "", "", "", ""], ["FEXT", "", "", "", "", "", "", ""]] caption="所有行"
  in  "Tap":T1(tab)
  out "开关型号":string
  in  "System_Mode":u16(ring) items=["A", "GPF001", "GPF002", "GPF003", "GPF004", "GPF005", "GPF006"]
  in  "Query":bool
  in  "Update":bool
  in  "Delete":bool
  in  "Save":bool
  in  "Local":bool
  in  "Luxshare_P/N:":string
  in  "Customer_P/N:":string
  in  "Customer":u16(ring) items=["Apple", "HuaWei", "HP", "Dell", "EMC", "Lenovo", "IBM", "Intel", "Inspur", "H3C", "MI", "Oppo", "Qlogics", "Others"]
  in  "Sample Description:":string
  in  "Cable AWG:":u16(ring) items=["24", "26", "28", "30", "32", "33"]
  in  "Length(mm):":string
  in  "Remark:":string
  in  "Excute":bool
  out "访问DB(s)":dbl format="%#_4g"
  out "仪器型号":string
  in  "ILD Spec":u16(ring) items=["IEEE802.3ba", "FDR", "EDR"]
  in  "Single Test Items":i32(listbox)
  in  "Diff Test Items":i32(listbox)
  in  "S-para Pair Name":i32(listbox)
  in  "NEXT Pair Name":i32(listbox)
  in  "FEXT Pair Name":i32(listbox)
  in  "VNA Cal File Path:":string="D:\\CALFILES\\"
  in  "Import Matrix?":bool caption="Start Test"
  out "Switch Matrix":string
  in  "Default":enum32{"Default", "Quick"}(radio)
  in  "TDR Test Items":i32(listbox)
  in  "Switch File Path":string="D:\\CALFILES\\"
  in  "Spec File Path":string="D:\\CALFILES\\"
  out "Spec _Data":dbl[][](array[numeric])
  in  "Spec Points":dbl=1601.0
  in  "Import Spec":bool caption="Start Test"
  in  "Spec Associate":string[][](table)
  in  "fre-save":string[](array[string]) caption="Save Frequency（MHZ）"
  in  "Default  fre":enum32{"Default", "Clear"}(radio)
  in  "Skew max(ps)":dbl=10.0
  in  "Impedance Spec:":string[][](table)=[["Mating Area", "1", "110", "1", "90"], ["Cable Area", "2", "105", "2", "95"]]
  in  "Impedance Filter":bool=TRUE
  in  "Filter Risetime(ps)":dbl=50.0 min=1.0 max=1000.0 step=1.0
  in  "StopTimeNs":dbl=5.0 min=1.0 max=100.0 step=0.1
  in  "Data Points":i32=4000 min=1000 max=10000 step=1
  in  "Compensation(ohm)":dbl=-3.0
  in  "Start TimeNs":dbl
  in  "Default":bool=TRUE
  in  "Quick":bool
  in  "Postion for \"PN&Tester&Date\" etc Fields":string[][](table)=[["Applicant", "0", "2", "1"], ["Part Name", "0", "3", "1"], ["Part Number", "0", "4", "1"], ["Report No", "0", "2", "12"], ["Sample No", "0", "4", "12"], ["Prepared By", "0", "63", "0"], ["Approved By", "0", "63", "6"], ["Date", "0", "63", "2"], ["Thru Result", "0", "13", "5"], ["NEXT Result", "0", "45", "4"], ["FEXT Result", "0", "45", "5"]]
  in  "Postion for Raw data":string[][](table)
  in  "Report Templete Path:":path
  in  "cancel dem2X?":bool
  out "Delay(ns)":dbl
  in  "From File":bool
  out "Delay":T2(graph)
  out "Insertion Loss":T2(graph)
  in  "Count(invisible)":string
  in  "FixtureType":string(combo)
  in  "FixtureNo":string(combo)
  in  "FixtureRev":string
  in  "Import_FixS4P":bool caption="Start Test"
  in  "Port Type":u16(ring)
  in  "YYWW":bool caption="每周更新SN"
  in  "AutoSN":bool
  in  "Label Num":string
  in  "Label Content":string
  in  "Label Print?":bool caption="Label Print ?"
  in  "EEPROM Write/Read ?":bool
  in  "SNType":string caption="SNFormat"
  in  "CmdType":u16(ring) caption="CableType" items=["", "Common_2X", "Common_1to4X", "H3C psw 10G_2X", "H3C psw 10G_1to4X", "H3C psw 28G_2X", "H3C psw 28G_1to4X"]
  # "SI Testing Project Management"
  # "2016/09/08  Rev1.2"
  # "(e.g. 40G ETHERNET QSFP+ to QSFP+ PASSIVE DAC CABLE)"
  # "(e.g.  D:\\CALFILES\\10G-AUTO-1601.csa)"
  # "Fre"
  # "1"
  # "2"
  # "3"
  # "4"
  # "5"
  # "6"
  # "7"
  # "8"
  # "9"
  # "10"
  # "保存频点请逐个加入，两个频点中间不要有空值！"
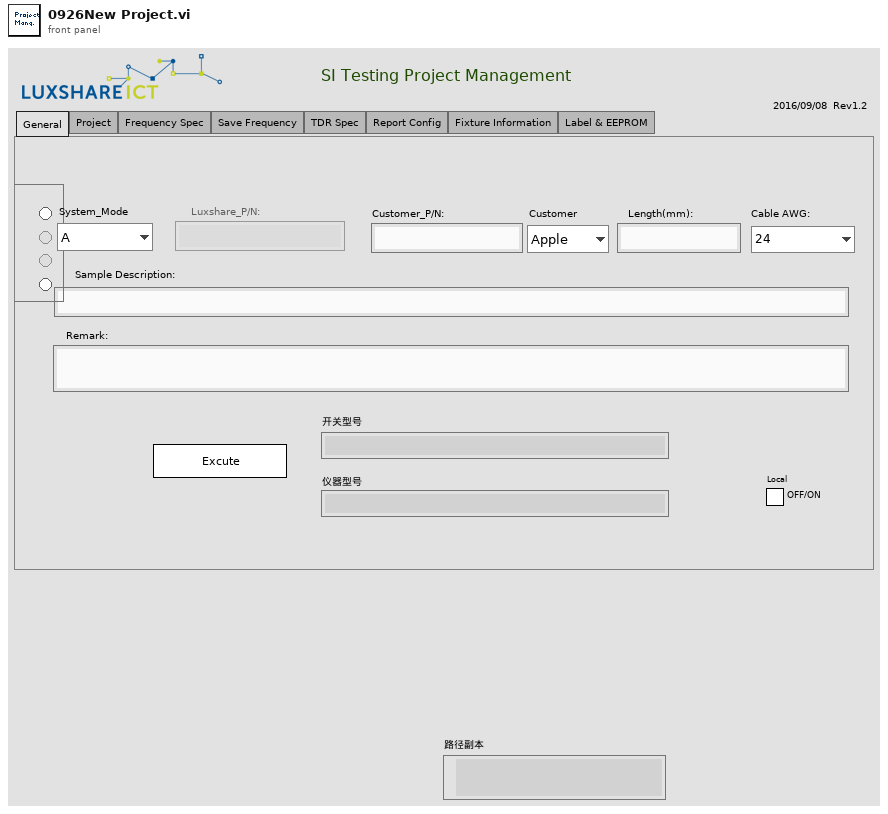
[diagram p1: front panel]
types:
  T1 = enum32{"General", "Project", "Frequency Spec", "Save Frequency", "TDR Spec", "Report Config", "Fixture Information", "Label & EEPROM"}
  T2 = cluster{"Frequency(Hz)":dbl[], "Diff S-parameters Data":dbl[]}
  T3 = typedef "LVRowAndColumnTypeDef.ctl" = cluster{"Row":i32, "Column":i32}
  T4 = enum8{"Enabled", "Disabled", "Disabled and Grayed Out"}
  T5 = typedef "LVComboBoxStrsAndValuesArrayTypeDef.ctl" = cluster{"String":string, "Value":string}[]
  T6 = enum16{"查询表名", "查询列名", "查询记录", "查询总记录", "查询数据", "转换数据"}
  T7 = enum16{"big-endian, network order", "native, host order", "little-endian"}
  T8 = enum16{"", "创建表", "删除表", "添加表列", "删除表列", "添加数据", "删除数据"}
  T9 = typedef "LVStringsAndValuesArrayTypeDef.ctl" = cluster{"String":string, "Value":u16}[]
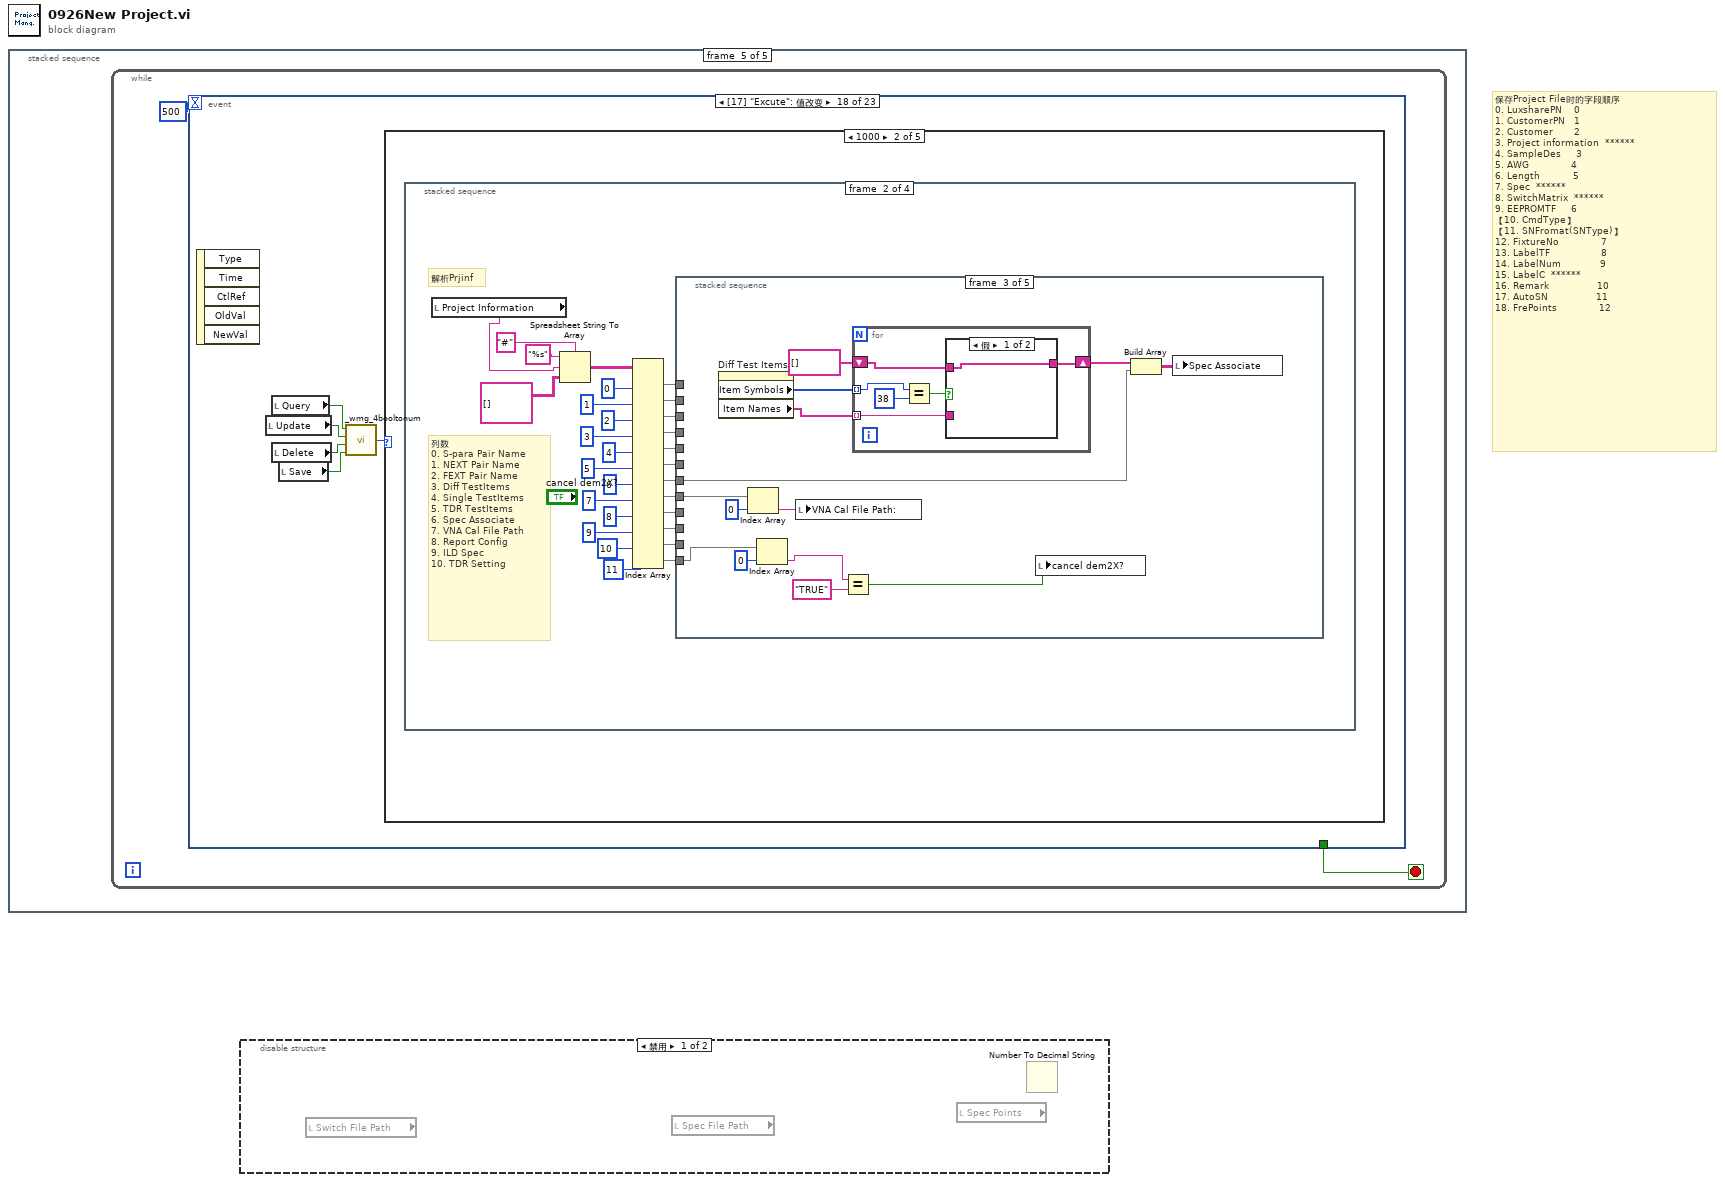
[diagram p0: block diagram]
diagram:
  # "保存Project File时的字段顺序\n0. LuxsharePN    0 \n1. CustomerPN   1\n2. Customer       2\n3. Project information  ****** \n4. SampleDes     3\n5. AWG              4\n6. Length           5\n7. Spec  ******\n8. SwitchMatrix  ******  \n9. EEPROMTF     6\n【10. CmdType】           \n【11. SNFromat(SNType)】   \n12. FixtureNo              7\n13. LabelTF                 8\n14. LabelNum             9\n15. LabelC  ******\n16. Remark                10\n17. AutoSN                11\n18. FrePoints              12"
  n1 = stacked-sequence {
    frame #0 {
      (unwired) string[][] [["Applicant", "0", "2", "1"], ["Part Name", "0", "3", "1"], ["Part Number", "0", "4", "1"], ["Report No", "0", "2", "12"], ["Sample No", "0", "4", "12"], ["Prepared By", "0", "63", "0"], ["Approved By", "0", "63", "6"], ["Date", "0", "63", "2"], ["Thru Result", "0", "13", "5"], ["NEXT Result", "0", "45", "4"], ["FEXT Result", "0", "45", "5"]] ("Postion for \"PN&Tester&Date\" etc Fields")
      w19 = T2 {"Frequency(Hz)"=[], "Diff S-parameters Data"=[]} ("输出簇")
      n2 = call <vilib>:"Application Directory.vi"() -> ("Application Directory"=w15:path)
      n3 = Build Path(base path=w15, name or relative path="Database" ("名称或相对路径")) -> (appended path=w13:path)
      n4 = call <vilib>:"Check if File or Folder Exists.vi"("path"=w13) -> ("file or folder exists?"=w12:bool, "dup path"=w11:path)  [unwired: 8 in, 1 out]
      n5 = case shown="假" w12 {
        tunnel: w11 -> [w22 w23]
        tunnel: [w21 w23] -> w10
        frame False {
          n6 = Create Folder(path (use dialog)=w22) -> (created path=w21:path)  [unwired: 2 in, 2 out]
        }
        frame True {
        }
      }
      n7 = Build Path(base path=w10, name or relative path="FigoConfig.xml" ("名称或相对路径")) -> (appended path=w8:path)
      n8 = call <vilib>:"Check if File or Folder Exists.vi"("path"=w8) -> ("dup path"=w7:path)  [unwired: 8 in, 2 out]
      "dup path" <- w7
      n9 = call "xmlConfigRead.vi"("path to XML document"=w7, "XPath expression"="//SystemList/NO/@Name") -> ("OutParaArray"=w3:string[])  [unwired: 2 out]
      n10 = call "xmlConfigRead.vi"("path to XML document"=w7, "XPath expression"="//SystemList/CurrentNO/@Name") -> ("OutParaArray"=w5:string[])  [unwired: 2 out]
      n11 = property on="Impedance Spec:" class="Tbl (严格)"("Active Cell"=T3 {"Row"=0, "Column"=0} ("活动单元格:活动单元格")) -> ()  [unwired: 2 in, 2 out]
      n12 = property on="System_Mode" class="Ring (严格)"("Strings []"=w3) -> ()  [unwired: 2 in, 2 out]
      n13 = property on="Import_FixS4P" class="Bool"("DisabledEnum"=2) -> ()  [unwired: 2 in, 2 out]
      n14 = local write "From File"(FALSE ("From File")) -> ()
      n15 = Index Array(array=w5, index=0 ("索引")) -> (element=w2:string)
      n16 = Search 1D Array(1D array=w3, element=w2) -> (index of element=w1:i32)  [unwired: 1 in]
      n17 = property on="System_Mode" class="Ring (严格)"("Val(Sgnl)"=w1) -> ()  [unwired: 2 in, 2 out]
      "Insertion Loss" <- w19
      "Delay" <- w19
    }
    frame #1 {
      w29 = T4."Disabled and Grayed Out" ("禁用")
      w41 = ""
      w57 = T3 {"Row"=0, "Column"=0} ("编辑位置")
      w58 = u32 4 ("列数")
      w59 = FALSE ("EEPROM Write/Read ?")
      w56 = 0 ("Diff Test Items")
      w61 = 37
      n18 = property on="Spec Associate" class="Tbl (严格)"("Number of Rows"=u32 2 ("行数")) -> ()  [unwired: 2 in, 2 out]
      n19 = call <vilib>:"Application Directory.vi"() -> ("Application Directory"=w88:path)
      n20 = local write "Switch Matrix"(w41) -> ()
      n21 = local write "Luxshare_P/N:"(w41) -> ()
      n22 = local write "Customer_P/N:"(w41) -> ()
      n23 = local write "Sample Description:"(w41) -> ()
      n24 = local write "Length(mm):"(w41) -> ()
      n25 = local write "Remark:"(w41) -> ()
      n26 = local write "Label Content"(w41) -> ()
      n27 = property on="Tap" class="TabCtl (严格)"("Value"=u32 0 ("行数")) -> ()  [unwired: 2 in, 2 out]
      n28 = Build Path(base path=w88, name or relative path="database\\inf.txt" ("名称或相对路径")) -> (appended path=w86:path)
      n29 = call-poly <vilib>:"Read From Spreadsheet File.vi"("file path (dialog if empty)"=w86) -> ("all rows"=w85:string[][])  [unwired: 6 in, 4 out]
      n30 = Delete From Array(array=w85, index (row)=0 ("索引 (行)")) -> (array with subset deleted=w66:string[][])  [unwired: 2 in, 1 out]
      "Inf" <- w66
      n31 = local write "VNA Cal File Path:"("D:\\CALFILES\\" ("VNA Cal File Path:")) -> ()
      n32 = Index Array(array=w66, index (col) #1=0 ("禁用的索引 (列)"), index (col) #2=1 ("索引 (列)"), index (col) #3=2 ("索引 (列)"), index (col) #4=3 ("索引 (列)"), index (col) #5=4 ("索引 (列)"), index (col) #6=5 ("索引 (列)")) -> (element #1=w78:string[], element #2=w77:string[], element #3=w76:string[], element #4=w75:string[], element #5=w74:string[], element #6=w63:string[])  [unwired: 6 in]
      n33 = call "Delete empty element from array.vi"("Array In"=w78) -> ("Array out"=w71:string[])  [unwired: 26 in]
      "Diff init" <- w71
      n34 = call "Delete empty element from array.vi"("Array In"=w77) -> ("Array out"=w38:string[])  [unwired: 26 in]
      "Single init" <- w38
      n35 = call "Delete empty element from array.vi"("Array In"=w76) -> ("Array out"=w37:string[])  [unwired: 26 in]
      "TDR init" <- w37
      n36 = call "Delete empty element from array.vi"("Array In"=w75) -> ("Array out"=w36:string[])  [unwired: 26 in]
      "S-p init" <- w36
      n37 = call "Delete empty element from array.vi"("Array In"=w74) -> ("Array out"=w35:string[])  [unwired: 26 in]
      "NEXT init" <- w35
      n38 = call "Delete empty element from array.vi"("Array In"=w63) -> ("Array out"=w34:string[])  [unwired: 26 in]
      "FEXT init" <- w34
      n39 = Array Size(array=w71) -> (size(s)=w92:i32)
      n40 = Array Size(array=w38) -> (size(s)=w89:i32)
      n41 = Array Size(array=w37) -> (size(s)=w62:i32)
      n42 = Array Size(array=w36) -> (size(s)=w72:i32)
      n43 = Array Size(array=w35) -> (size(s)=w90:i32)
      n44 = Array Size(array=w34) -> (size(s)=w73:i32)
      n45 = property on="Postion for Raw data" class="Tbl (严格)"("Value"=string[][] [] ("Postion for Raw data")) -> ()  [unwired: 2 in, 2 out]
      n46 = Initialize Array(w61, w92) -> (w53:i32[])
      "Diff init" <- w53
      n47 = Initialize Array(w61, w89) -> (w52:i32[])
      "Single init" <- w52
      n48 = Initialize Array(w61, w62) -> (w51:i32[])
      "TDR init" <- w51
      n49 = Initialize Array(w61, w72) -> (w91:i32[])
      "S-p init" <- w91
      n50 = Initialize Array(w61, w90) -> (w50:i32[])
      "NEXT init" <- w50
      n51 = Initialize Array(w61, w73) -> (w49:i32[])
      "FEXT init" <- w49
      n52 = property on="Diff Test Items" class="LstBox (严格)"("Item Names"=w71, "Item Symbols"=w53) -> ()  [unwired: 2 in, 2 out]
      n53 = property on="Single Test Items" class="LstBox (严格)"("Item Names"=w38, "Item Symbols"=w52) -> ()  [unwired: 2 in, 2 out]
      n54 = property on="TDR Test Items" class="LstBox (严格)"("Item Names"=w37, "Item Symbols"=w51) -> ()  [unwired: 2 in, 2 out]
      n55 = property on="S-para Pair Name" class="LstBox (严格)"("Item Names"=w36, "Item Symbols"=w91) -> ()  [unwired: 2 in, 2 out]
      n56 = property on="NEXT Pair Name" class="LstBox (严格)"("Item Names"=w35, "Item Symbols"=w50) -> ()  [unwired: 2 in, 2 out]
      n57 = property on="FEXT Pair Name" class="LstBox (严格)"("Item Names"=w34, "Item Symbols"=w49) -> ()  [unwired: 2 in, 2 out]
      n58 = property on="访问DB(s)" class="DigNum (严格)"("Visible"=TRUE ("可见")) -> ()  [unwired: 2 in, 2 out]
      n59 = local write "fre-save"(string[] [] ("fre-save")) -> ()
      n60 = Get Date/Time In Seconds() -> (seconds since 1Jan1904=→"midVar_timeStart":timestamp)
      n61 = local write "EEPROM Write/Read ?"(w59) -> ()
      n62 = local write "Report Templete Path:"(path "" ("Report Templete Path:")) -> ()
      n63 = local write "Label Print?"(w59) -> ()
      n64 = property on="Postion for Raw data" class="Tbl (严格)"("Number of Columns"=w58, "EditPos"=w57) -> ()  [unwired: 2 in, 2 out]
      n65 = property on="Postion for \"PN&Tester&Date\" etc Fields" class="Tbl (严格)"("Number of Columns"=w58, "EditPos"=w57) -> ()  [unwired: 2 in, 2 out]
      n66 = property on="Postion for \"PN&Tester&Date\" etc Fields" class="Tbl (严格)"("Value"=string[][] [["Applicant", "0", "2", "1"], ["Part Name", "0", "3", "1"], ["Part Number", "0", "4", "1"], ["Report No", "0", "2", "12"], ["Sample No", "0", "4", "12"], ["Prepared By", "0", "63", "0"], ["Approved By", "0", "63", "6"], ["Date", "0", "63", "2"], ["Thru Result", "0", "13", "5"], ["NEXT Result", "0", "45", "4"], ["FEXT Result", "0", "45", "5"]] ("Postion for \"PN&Tester&Date\" etc Fields")) -> ()  [unwired: 2 in, 2 out]
      n67 = local write "Spec Points"(1601.0 ("Spec Points")) -> ()
      n68 = local write "Quick"(FALSE ("Quick")) -> ()
      n69 = local write "Spec _Data"(dbl[][] [] ("添加的数组")) -> ()
      n70 = property on="Spec Associate" class="Tbl (严格)"("Value"=string[][] [] ("已删除元素的数组子集")) -> ()  [unwired: 2 in, 2 out]
      n71 = property on="Diff Test Items" class="LstBox (严格)"("Value"=w56) -> ()  [unwired: 2 in, 2 out]
